vi "Drive Immediate.vi"(7 "Description":string, 8 "Command Info In":T1, 9 "Deadband Value":dbl=0.05, 10 "Right Setpoint":dbl, 11 "Left Setpoint":dbl) -> (0 "Command Info Out":T1)   [LabVIEW 2018]
doc: "Often used for joystick control, this VI checks to see that the joystick axes are outside the deadband and updates the motors appropriately."
uses:
  <vilib>/Rock Robotics/WPI/Framework/Command Status Info.ctl
  <vilib>/Rock Robotics/WPI/Framework/Completion Status.ctl
  <vilib>/Rock Robotics/WPI/Framework/Completion Notifier.ctl
  Implementation/Drive Setpoints.ctl
  Implementation/Drive Operations.ctl
  <vilib>/ptbypt/NI_PtbyPt.lvlib
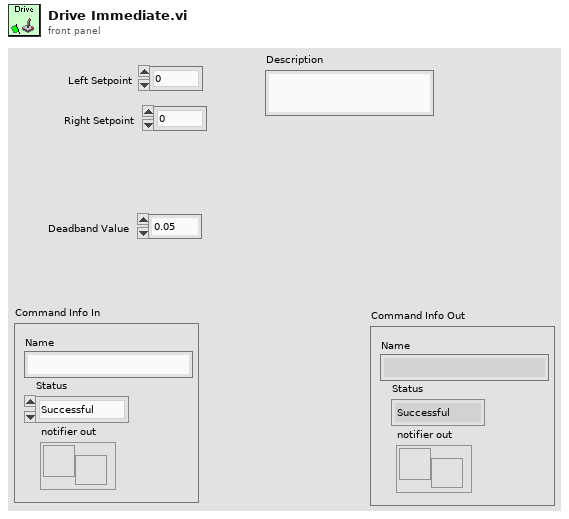
[diagram p1: front panel]
types:
  T1 = typedef "Command Status Info.ctl" = cluster{"Name":string, "Status":T2, "notifier out":T3}
  T2 = typedef "Completion Status.ctl" = enum16{"Successful", "Aborted", "Incomplete"}
  T3 = typedef "Completion Notifier.ctl" = refnum<notifier>
  T4 = typedef "Drive Setpoints.ctl" = cluster{"Operation":T5, "Left Setpoint":dbl, "Right Setpoint":dbl, "Duration":dbl, "Distance":dbl, "Target Angle":dbl, "Speed":dbl}
  T5 = typedef "Drive Operations.ctl" = enum16{"Reserve", "Read Current", "Immediate", "Drive for Time", "Drive for Distance", "Drive Distance Line", "Drive to Angle Relative", "Drive to Angle", "Run Motion Profile", "Auto Turn", "Reset Encoders", "Reset Gyro"}
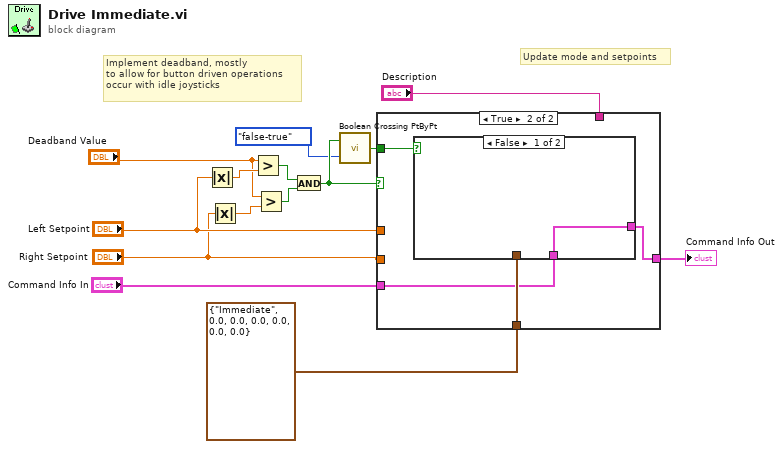
[diagram p0: block diagram]
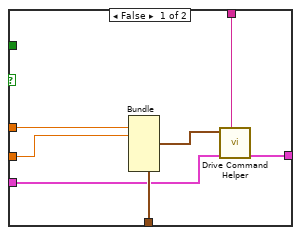
[diagram p2: hidden frame]
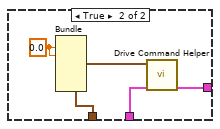
[diagram p3: hidden frame]
diagram:
  # "Implement deadband, mostly\nto allow for button driven operations\noccur with idle joysticks"
  # "Update mode and setpoints"
  n1 = Absolute Value(x="Left Setpoint") -> (abs(x)=w14:dbl)
  n2 = Absolute Value(x="Right Setpoint") -> (abs(x)=w7:dbl)
  n3 = Greater?(x="Deadband Value", y=w14) -> (0:w8:bool)
  n4 = Greater?(x="Deadband Value", y=w7) -> (0:w5:bool)
  n5 = And(x=w8, y=w5) -> (x .and. y?=w3:bool)
  n6 = call <vilib>:"Boolean Crossing PtByPt.vi"("direction"=enum16{"either", "false-true", "true-false"}."false-true", "input"=w3) -> ("crossing"=w2:bool)  [unwired: 1 in]
  n7 = case shown="True" w3 {
    tunnel: "Left Setpoint" -> [w21 _]
    tunnel: T4 {"Operation"=enum."Immediate", "Left Setpoint"=0.0, "Right Setpoint"=0.0, "Duration"=0.0, "Distance"=0.0, "Target Angle"=0.0, "Speed"=0.0} ("SubSystem Data") -> [w20 w24]
    tunnel: [w19 w22] -> w13
    tunnel: "Command Info In" -> [w18 w23]
    tunnel: "Description" -> [w16 _]
    tunnel: "Right Setpoint" -> [w15 _]
    tunnel: w2 -> [_ w25]
    frame False {
      n8 = Bundle(cluster=w20, "Left Setpoint"=w21, "Right Setpoint"=w15) -> (w17:T4)  [unwired: 5 in]
      n9 = call "Drive Command Helper.vi"("Description"=w16, "Command Info In"=w18, "SubSystem Data"=w17) -> ("Command Info Out"=w19:T1)  [unwired: 6 in, 2 out]
    }
    frame True {
      n10 = case shown="False" w25 {
        tunnel: w24 -> [_ w30]
        tunnel: w23 -> [w26 w28]
        tunnel: [w26 w27] -> w22
        frame False {
        }
        frame True {
          w29 = 0.0 ("Left Setpoint")
          n11 = Bundle(cluster=w30, "Left Setpoint"=w29, "Right Setpoint"=w29) -> (w31:T4)  [unwired: 5 in]
          n12 = call "Drive Command Helper.vi"("Command Info In"=w28, "SubSystem Data"=w31) -> ("Command Info Out"=w27:T1)  [unwired: 7 in, 2 out]
        }
      }
    }
  }
  "Command Info Out" <- w13
